vi "GSP_GUI_ComponentLoad.vi"(4 "error in (no error)":errorcluster, 6 "Old Component List":T1, 7 "New Component List":T1) -> (0 "error out":errorcluster, 2 "Changes complete?":bool)   [LabVIEW 2015]
uses:
  Systems/SystemUtil/ComponentList.ctl
  Systems/Slit/slitactions.ctl
  GSP_GUI_global.vi
panel:
  out "Message":string
  out "Old":string
  out "New":string
  out "System":string
  in  "Script#":i32
  in  "Next":bool
  # "Systems will automatically move the\ncomponent to be added/removed into\nthe corresponding load position.\n\nPerform the operation displayed to the\nright.  Hitting next verifies the action\nhas been completed"
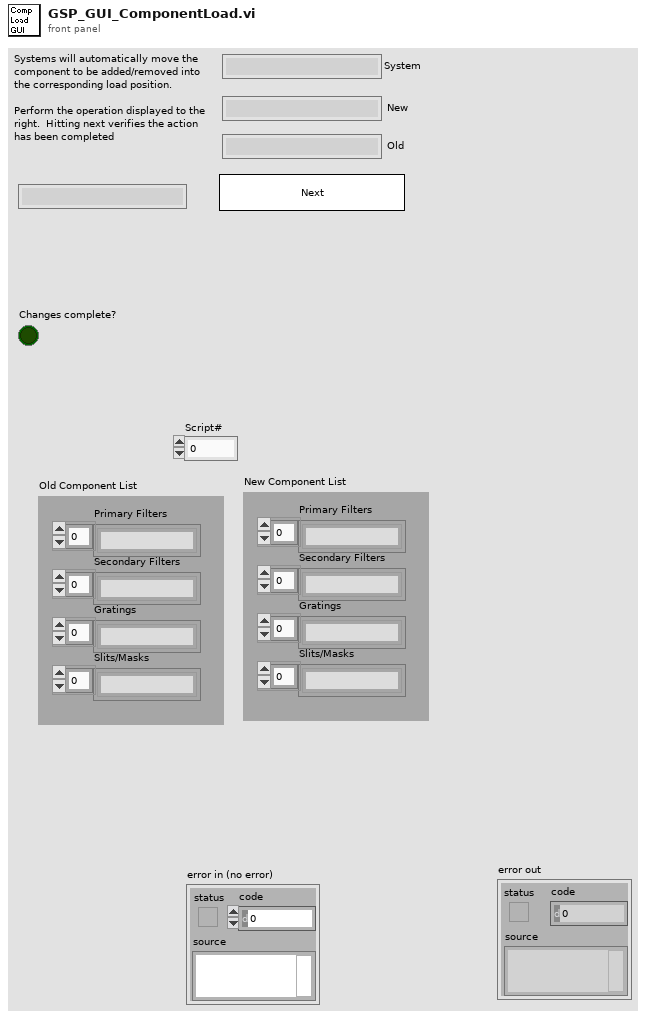
[diagram p1: front panel]
types:
  T1 = typedef "ComponentList.ctl" = cluster{"Primary Filters":string[], "Secondary Filters":string[], "Gratings":string[], "Slits/Masks":string[]}
  T2 = cluster{"Component Type":enum16{"primary filter", "secondary filter", "grating", "slit/mask"}, "Component#":i32, "Old Component":string, "New Component":string}[]
  T3 = enum16{"Launch", "INIT_CTL", "Home", "Move", "Shutdown"}
  T4 = enum16{"Launch", "INIT_CTL", "Move", "Home", "Shutdown"}
  T5 = typedef "slitactions.ctl" = enum16{"Launch", "INIT_CTL", "Restart", "Show", "Hide", "Home", "Move", "Rotate Only", "Shutdown"}
  T6 = cluster{"Component Type":enum16{"primary filter", "secondary filter", "grating", "slit/mask"}, "Component#":i32, "Old Component":string, "New Component":string}
  T7 = enum16{"primary filter", "secondary filter", "grating", "slit/mask"}
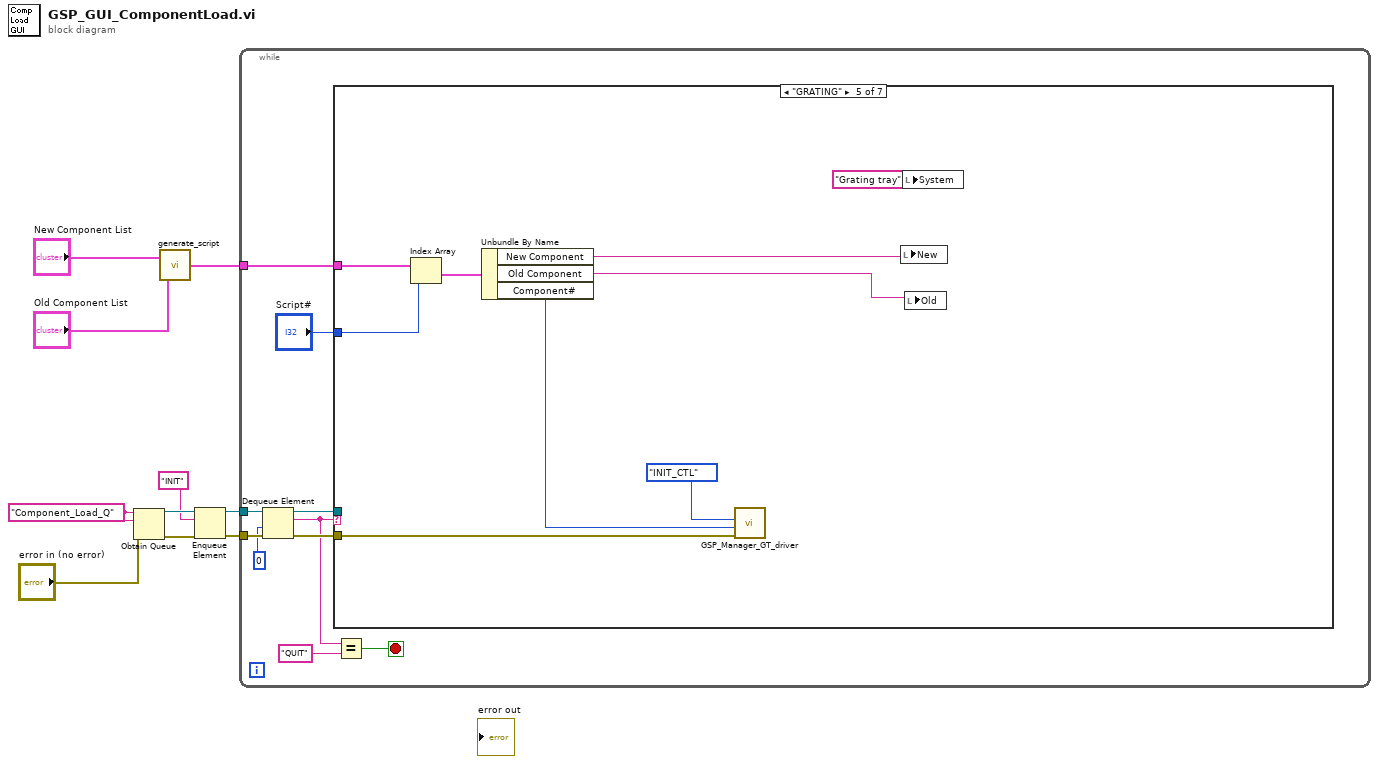
[diagram p0: block diagram]
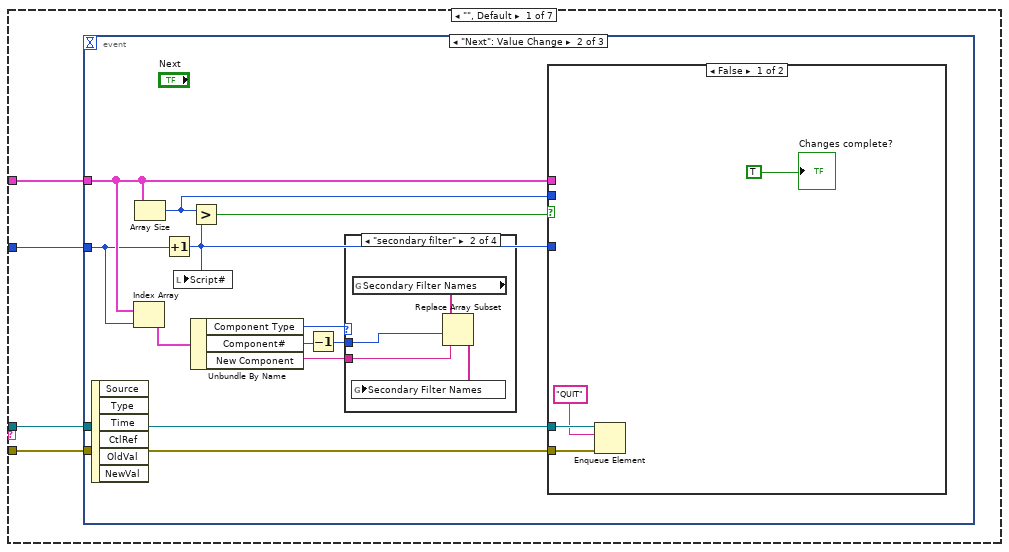
[diagram p2: hidden frame]
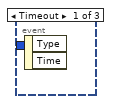
[diagram p3: hidden frame]
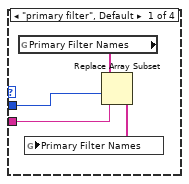
[diagram p4: hidden frame]
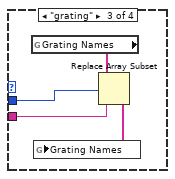
[diagram p5: hidden frame]
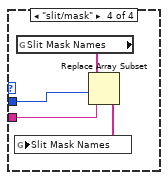
[diagram p6: hidden frame]
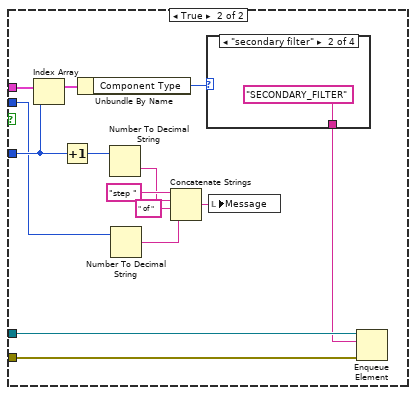
[diagram p7: hidden frame]
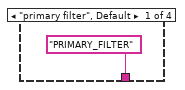
[diagram p8: hidden frame]
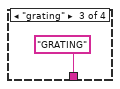
[diagram p9: hidden frame]
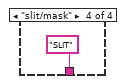
[diagram p10: hidden frame]
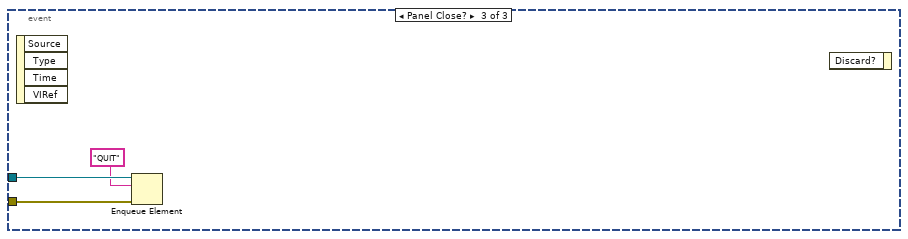
[diagram p11: hidden frame]
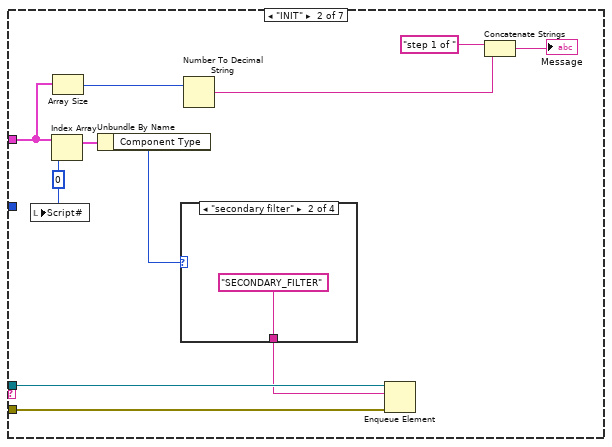
[diagram p12: hidden frame]
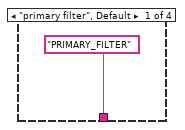
[diagram p13: hidden frame]
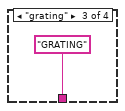
[diagram p14: hidden frame]
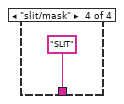
[diagram p15: hidden frame]
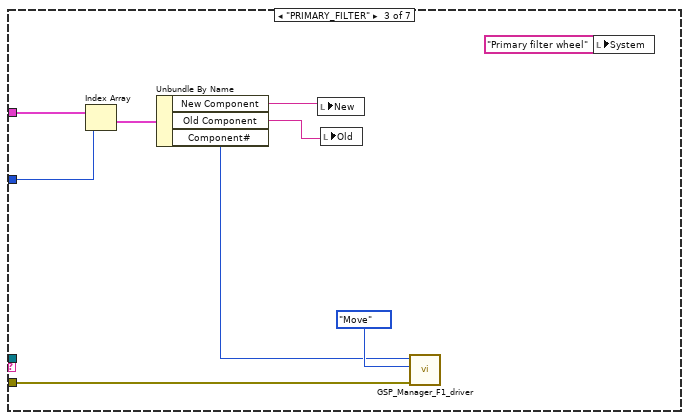
[diagram p16: hidden frame]
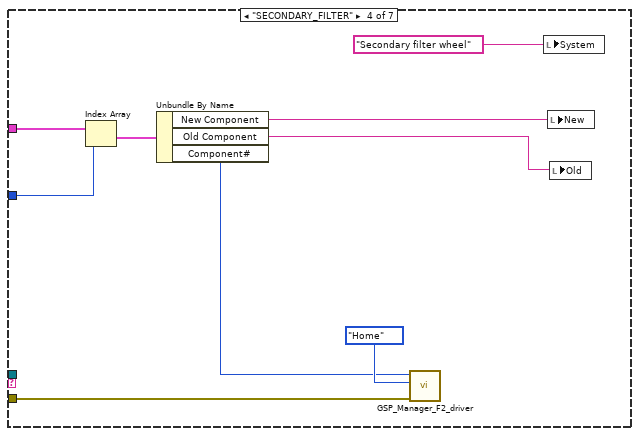
[diagram p17: hidden frame]
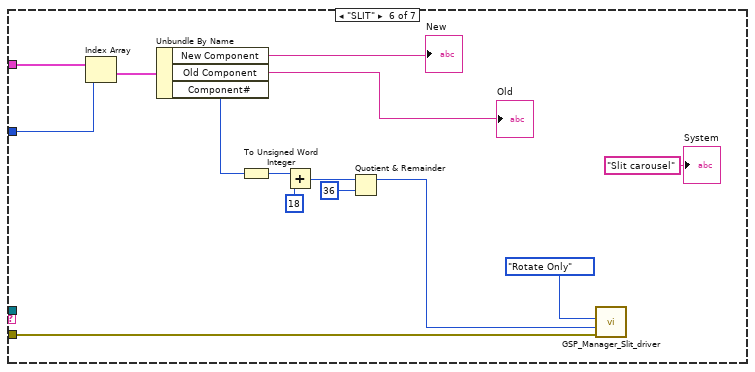
[diagram p18: hidden frame]
diagram:
  w6 = "Component_Load_Q" ("name (unnamed)")
  n1 = Obtain Queue(name (unnamed)=w6, element data type=w6, error in (no error)="error in (no error)") -> (queue out=w8:refnum<queue>, error out=w7:errorcluster)  [unwired: 2 in, 1 out]
  n2 = call "generate_script.vi"("Old Component List"="Old Component List", "New Component List"="New Component List") -> ("Component Change Script"=w1:T2)
  n3 = Enqueue Element(queue=w8, element="INIT", error in (no error)=w7) -> (queue out=w3:refnum<queue>, error out=w2:errorcluster)  [unwired: 1 in, 1 out]
  n4 = while {
    tunnel: w3 -> [w20]
    tunnel: w2 -> [w19]
    tunnel: w1 -> [w12]
    stop <- w14 stop-if-true
    n5 = Dequeue Element(queue=w20, timeout in ms (-1)=0, error in (no error)=w19) -> (queue out=w18:refnum<queue>, element=w16:string, error out=w17:errorcluster)  [unwired: 1 out]
    n6 = case shown="\"GRATING\"" w16 {
      tunnel: w18 -> [w23 w88 _ _ _ _ _]
      tunnel: w17 -> [w24 w87 w101 w110 w119 w133 _]
      tunnel: w12 -> [w22 w81 w99 w108 w118 w132 _]
      tunnel: "Script#" -> [w21 _ w98 w107 w117 w131 _]
      frame "", Default {
        n7 = event shown="[1] \"Next\": Value Change" {
          selector: _ -> [_ _ _]
          dyn-events: _ -> [_ _ _]
          timeout: _ -> [_ _ _]
          tunnel: w24 -> [_ w34 w76]
          tunnel: w23 -> [_ w35 w77]
          tunnel: w22 -> [_ w32 _]
          tunnel: w21 -> [_ w31 _]
          event Timeout {
            n8 = event-data() -> ()  [unwired: 1 in, 2 out]
          }
          event "Next": Value Change {
            n9 = event-data() -> ()  [unwired: 1 in, 6 out]
            n10 = Index Array(array=w32, index=w31) -> (element=w26:T6)
            n11 = Array Size(array=w32) -> (size(s)=w25:i32)
            n12 = Increment(x=w31) -> (x+1=w33:i32)
            n13 = local write "Script#"(w33) -> ()
            n14 = Greater?(x=w25, y=w33) -> (0:w36:bool)
            n15 = Unbundle By Name(w26) -> ("Component Type"=w28:T7, "Component#"=w27:i32, "New Component"=w30:string)
            n16 = Decrement(x=w27) -> (x-1=w29:i32)
            n17 = case shown="\"secondary filter\"" w28 {
              tunnel: w29 -> [w38 w42 w46 w50]
              tunnel: w30 -> [w37 w41 w45 w49]
              frame "primary filter", Default {
                n18 = global read "GSP_GUI_global.vi" "Primary Filter Names"() -> (w40:string[])
                n19 = Replace Array Subset(array=w40, new element=w37, index=w38) -> (w39:string[])
                n20 = global write "GSP_GUI_global.vi" "Primary Filter Names"(w39) -> ()
              }
              frame "secondary filter" {
                n21 = global read "GSP_GUI_global.vi" "Secondary Filter Names"() -> (w44:string[])
                n22 = Replace Array Subset(array=w44, new element=w41, index=w42) -> (w43:string[])
                n23 = global write "GSP_GUI_global.vi" "Secondary Filter Names"(w43) -> ()
              }
              frame "grating" {
                n24 = global read "GSP_GUI_global.vi" "Grating Names"() -> (w48:string[])
                n25 = Replace Array Subset(array=w48, new element=w45, index=w46) -> (w47:string[])
                n26 = global write "GSP_GUI_global.vi" "Grating Names"(w47) -> ()
              }
              frame "slit/mask" {
                n27 = global read "GSP_GUI_global.vi" "Slit Mask Names"() -> (w52:string[])
                n28 = Replace Array Subset(array=w52, new element=w49, index=w50) -> (w51:string[])
                n29 = global write "GSP_GUI_global.vi" "Slit Mask Names"(w51) -> ()
              }
            }
            n30 = case shown="False" w36 {
              tunnel: w35 -> [w56 w68]
              tunnel: w34 -> [w55 w67]
              tunnel: w32 -> [_ w70]
              tunnel: w33 -> [_ w64]
              tunnel: w25 -> [_ w59]
              frame False {
                n31 = Enqueue Element(queue=w56, element="QUIT", error in (no error)=w55) -> ()  [unwired: 1 in, 3 out]
                "Changes complete?" <- TRUE
              }
              frame True {
                n32 = Index Array(array=w70, index=w64) -> (element=w69:T6)
                n33 = Increment(x=w64) -> (x+1=w63:i32)
                n34 = Unbundle By Name(w69) -> ("Component Type"=w65:T7)
                n35 = Number To Decimal String(number=w63) -> (decimal integer string=w61:string)  [unwired: 1 in]
                n36 = Number To Decimal String(number=w59) -> (decimal integer string=w58:string)  [unwired: 1 in]
                n37 = Concatenate Strings("step ", w61, " of " ("string"), w58) -> (w57:string)
                n38 = case shown="\"secondary filter\"" w65 {
                  tunnel: ["PRIMARY_FILTER" "SECONDARY_FILTER" "GRATING" "SLIT"] -> w66
                  frame "primary filter", Default {
                  }
                  frame "secondary filter" {
                  }
                  frame "grating" {
                  }
                  frame "slit/mask" {
                  }
                }
                n39 = local write "Message"(w57) -> ()
                n40 = Enqueue Element(queue=w68, element=w66, error in (no error)=w67) -> ()  [unwired: 1 in, 3 out]
              }
            }
          }
          event Panel Close? {
            n41 = event-data() -> ()  [unwired: 1 in, 4 out]
            n42 = Enqueue Element(queue=w77, element="QUIT", error in (no error)=w76) -> ()  [unwired: 1 in, 3 out]
            n43 = event-data() -> ()  [unwired: 2 in, 1 out]
          }
        }
      }
      frame "INIT" {
        w83 = 0
        n44 = local write "Script#"(w83) -> ()
        n45 = Index Array(array=w81, index=w83) -> (element=w86:T6)
        n46 = Array Size(array=w81) -> (size(s)=w80:i32)
        n47 = Unbundle By Name(w86) -> ("Component Type"=w85:T7)
        n48 = case shown="\"secondary filter\"" w85 {
          tunnel: ["PRIMARY_FILTER" "SECONDARY_FILTER" "GRATING" "SLIT"] -> w84
          frame "primary filter", Default {
          }
          frame "secondary filter" {
          }
          frame "grating" {
          }
          frame "slit/mask" {
          }
        }
        n49 = Number To Decimal String(number=w80) -> (decimal integer string=w79:string)  [unwired: 1 in]
        n50 = Enqueue Element(queue=w88, element=w84, error in (no error)=w87) -> ()  [unwired: 1 in, 3 out]
        n51 = Concatenate Strings("step 1 of ", w79) -> (→"Message":string)
      }
      frame "PRIMARY_FILTER" {
        n52 = Index Array(array=w99, index=w98) -> (element=w97:T6)
        n53 = Unbundle By Name(w97) -> ("New Component"=w94:string, "Old Component"=w93:string, "Component#"=w96:i32)
        n54 = local write "New"(w94) -> ()
        n55 = local write "Old"(w93) -> ()
        n56 = call "GSP_Manager_F1_driver.vi"("error in (no error)"=w101, "Action"=T3."Move", "Filter# (Move Only)"=w96) -> ()  [unwired: 3 in, 2 out]
        n57 = local write "System"("Primary filter wheel" ("System")) -> ()
      }
      frame "SECONDARY_FILTER" {
        n58 = Index Array(array=w108, index=w107) -> (element=w106:T6)
        n59 = Unbundle By Name(w106) -> ("New Component"=w103:string, "Old Component"=w102:string, "Component#"=w105:i32)
        n60 = call "GSP_Manager_F2_driver.vi"("error in (no error)"=w110, "Action"=T3."Home", "Filter# (Move Only)"=w105) -> ()  [unwired: 3 in, 2 out]
        n61 = local write "System"("Secondary filter wheel" ("System")) -> ()
        n62 = local write "New"(w103) -> ()
        n63 = local write "Old"(w102) -> ()
      }
      frame "GRATING" {
        n64 = Index Array(array=w118, index=w117) -> (element=w116:T6)
        n65 = Unbundle By Name(w116) -> ("New Component"=w112:string, "Old Component"=w111:string, "Component#"=w115:i32)
        n66 = call "GSP_Manager_GT_driver.vi"("error in (no error)"=w119, "Grating # (Move Only)"=w115, "Action"=T4."INIT_CTL") -> ()  [unwired: 3 in, 2 out]
        n67 = local write "New"(w112) -> ()
        n68 = local write "System"("Grating tray" ("System")) -> ()
        n69 = local write "Old"(w111) -> ()
      }
      frame "SLIT" {
        n70 = Index Array(array=w132, index=w131) -> (element=w130:T6)
        n71 = Unbundle By Name(w130) -> ("New Component"=→"New":string, "Old Component"=→"Old":string, "Component#"=w129:i32)
        n72 = To Unsigned Word Integer(number=w129) -> (unsigned 16bit integer=w124:u16)
        n73 = Add(x=w124, y=u16 18) -> (x+y=w122:u16)
        n74 = Quotient & Remainder(x=w122, y=u16 36) -> (x-y*floor(x/y)=w120:u16)  [unwired: 1 out]
        n75 = call "GSP_Manager_Slit_driver.vi"("error in (no error)"=w133, "Slit # (Move/Rotate Only)"=w120, "Action"=slitactions."Rotate Only") -> ()  [unwired: 3 in, 2 out]
        "System" <- "Slit carousel" ("System")
      }
      frame "QUIT" {
      }
    }
    n76 = Equal?(x=w16, y="QUIT") -> (x = y?=w14:bool)
  }
